vi "Translate Color.vi"(11 "color string":string) -> (2 "dark?":bool, 3 "color":u32(colorbox))   [LabVIEW 2017]
doc: "Converts <b>color string</b> into appropriate numeric value and informs if the color is dark."
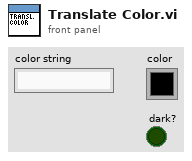
[diagram p1: front panel]
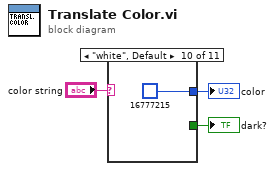
[diagram p0: block diagram]
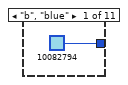
[diagram p2: hidden frame]
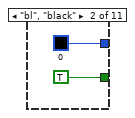
[diagram p3: hidden frame]
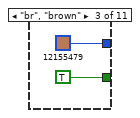
[diagram p4: hidden frame]
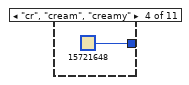
[diagram p5: hidden frame]
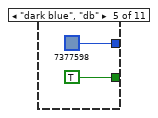
[diagram p6: hidden frame]
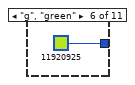
[diagram p7: hidden frame]
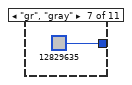
[diagram p8: hidden frame]
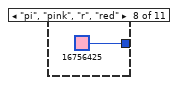
[diagram p9: hidden frame]
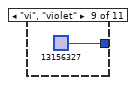
[diagram p10: hidden frame]
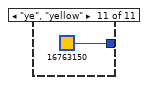
[diagram p11: hidden frame]
diagram:
  n1 = case shown="\"white\", Default" "color string" {
    tunnel: [u32 10082794 ("color(white)") u32 0 ("color(white)") u32 12155479 ("color(white)") u32 15721648 ("color(white)") u32 7377598 ("color(white)") u32 11920925 ("color(white)") u32 12829635 ("color(white)") u32 16756425 ("color(white)") u32 13156327 ("color(white)") u32 16777215 ("color(white)") u32 16763150 ("color(white)")] -> w1
    tunnel: [_ TRUE TRUE _ TRUE _ _ _ _ _ _] -> w2
    frame "b", "blue" {
    }
    frame "bl", "black" {
    }
    frame "br", "brown" {
    }
    frame "cr", "cream", "creamy" {
    }
    frame "dark blue", "db" {
    }
    frame "g", "green" {
    }
    frame "gr", "gray" {
    }
    frame "pi", "pink", "r", "red" {
    }
    frame "vi", "violet" {
    }
    frame "white", Default {
    }
    frame "ye", "yellow" {
    }
  }
  "dark?" <- w2
  "color" <- w1
